vi "testB.vi"(10 "Internal B":refnum<vi>, 11 "Commande numérique 2":i32) -> (3 "Commande numérique":i32)   [LabVIEW 2016]
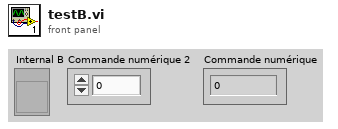
[diagram p1: front panel]
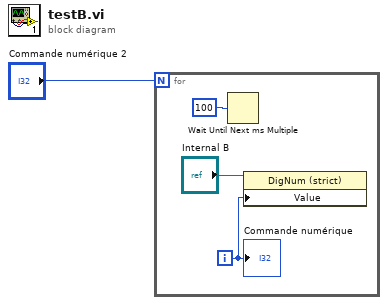
[diagram p0: block diagram]
diagram:
  n1 = for {
    N: "Commande numérique 2" -> [_]
    i -> [w2]
    n2 = Wait Until Next ms Multiple(millisecond multiple=u32 100 ("n millisecondes")) -> ()  [unwired: 1 out]
    n3 = property class="DigNum (strict)"(reference="Internal B", "Value"=w2) -> ()  [unwired: 1 in, 2 out]
    "Commande numérique" <- w2
  }
